vi "Serialize - JSON.vi"(8 "error in":errorcluster, 11 "M data in":refnum<class "M data.lvclass">) -> (0 "error out":errorcluster, 2 "Serialized JSON":string, 3 "M data out":refnum<class "M data.lvclass">)   [LabVIEW 2015, in "Alicat Lib.lvlib" / "M data.lvclass"]
uses:
  M data.lvclass
  M data.lvclass/M data.ctl
  Alicat Data.lvclass
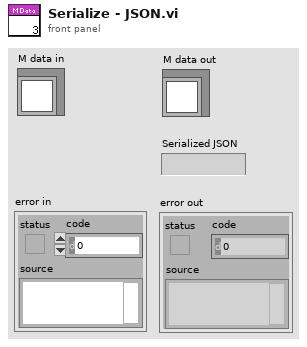
[diagram p1: front panel]
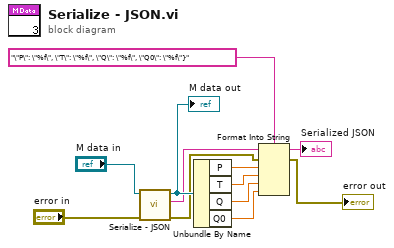
[diagram p0: block diagram]
diagram:
  n1 = call-parent "Serialize - JSON.vi"("error in"="error in", "Alicat Data in"="M data in") -> ("error out"=w2:errorcluster, "Serialized JSON"=w9:string, "Alicat Data out"=w10:refnum<class "M data.lvclass">)  [unwired: 7 in]
  "M data out" <- w10
  n2 = Unbundle By Name(w10) -> ("P"=w6:sgl, "T"=w5:sgl, "Q"=w4:sgl, "Q0"=w3:sgl)
  n3 = Format Into String(format string="\"P\": \"%f\", \"T\": \"%f\", \"Q\": \"%f\", \"Q0\": \"%f\"}", initial string=w9, error in=w2, w6, w5, w4, w3) -> (resulting string=→"Serialized JSON":string, error out=→"error out":errorcluster)
